vi "Set FP Items.vi"(7 "VI Ref":refnum<vi>, 8 "Error":errorcluster, 11 "FPEN":refnum<class "FPEN.lvclass">) -> (0 "Error Out":errorcluster, 3 "FPEN Out":refnum<class "FPEN.lvclass">, 5 "VI Ref Out":refnum<vi>)   [LabVIEW 2025, in "FPEN.lvclass"]
uses:
  FPEN.lvclass
  FPEN.lvclass/FPEN.ctl
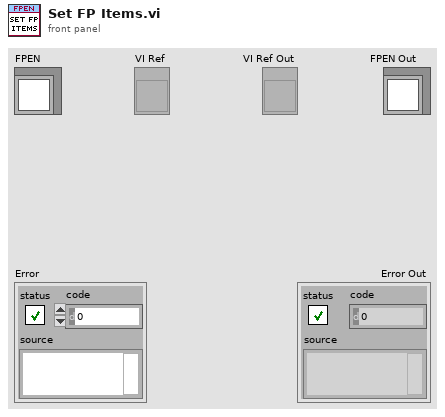
[diagram p1: front panel]
types:
  T1 = typedef "Cluster_FP_Scroll Bars Hide Show.ctl" = cluster{"Horiz SBar":T2, "Vert SBar":T2}
  T2 = typedef "ENUM_FP_Show-Hide Select.ctl" = enum16{"No Change", "Hide", "Show"}
  T3 = typedef "Cluster_FP_Show Hide Items.ctl" = cluster{"MenuBar":T2, "FreeRunButton":T2, "RunButton":T2, "AbortButton":T2, "ToolBar":T2, "Resize":T2, "Closeable":T2, "Minimizable":T2}
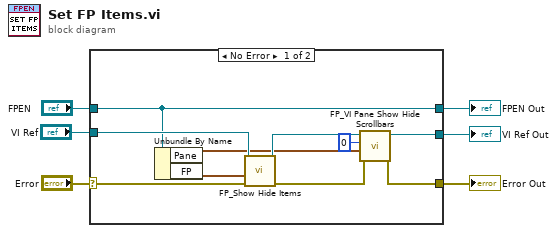
[diagram p0: block diagram]
diagram:
  n1 = case shown="No Error" "Error" {
    selector: "Error" -> [w14 w19]
    tunnel: [w9 w19] -> w5
    tunnel: [w13 w18] -> w3
    tunnel: "FPEN" -> [w13 w18]
    tunnel: [w11 w17] -> w2
    tunnel: "VI Ref" -> [w15 w17]
    frame No Error {
      n2 = Unbundle By Name(w13) -> ("Pane"=w8:T1, "FP"=w16:T3)
      n3 = call "FP_Show Hide Items.vi"("Error"=w14, "FP Show Hide"=w16, "VI"=w15) -> ("Error Out"=w10:errorcluster, "VI Out"=w12:refnum<vi>)  [unwired: 7 in]
      n4 = call "FP_VI Pane Show Hide Scrollbars.vi"("Error"=w10, "Scrollbar Settings"=w8, "Pane Index"=0, "VI"=w12) -> ("Error Out"=w9:errorcluster, "VI Out"=w11:refnum<vi>)  [unwired: 6 in]
    }
    frame Error {
    }
  }
  "Error Out" <- w5
  "FPEN Out" <- w3
  "VI Ref Out" <- w2
